vi "SimpleRegAndResolve.vi"() -> ()   [LabVIEW 2024, in "Module Container.lvlib"]
uses:
  Module Container.lvlib
  ModuleTemplates/NewTemplateModule/NewTemplate.lvclass
  C:/Git/JA/JQMH/RQMHCore/ModuleCore/Module.lvclass
  C:/Git/JA/JQMH/ModuleTemplates/NewTemplateModule/NewTemplate.lvclass
  ModuleCore/Module.lvclass
  Startup/ModuleStartup.lvclass
panel:
  out "Already Running":bool
  out "error out":errorcluster
  in  "stop":bool
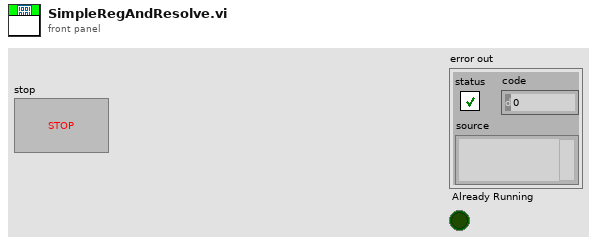
[diagram p1: front panel]
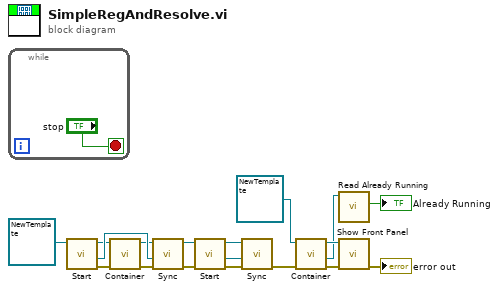
[diagram p0: block diagram]
diagram:
  n1 = while {
    stop <- "stop" stop-if-true
  }
  n2 = call "Start.vi"("JQMHCore in"=refnum<class "NewTemplate.lvclass"> refnum ("Template")) -> ("error out"=w9:errorcluster, "StartupHandshake out"=w18:refnum<class "ModuleStartup.lvclass">, "JQMHCore out"=w13:refnum<class "NewTemplate.lvclass">)  [unwired: 8 in]
  n3 = call "Container.vi"("error in (no error)"=w9, "Module Type"=w13) -> ("error out"=w8:errorcluster, "Module Instance"=w12:refnum<class "NewTemplate.lvclass">)  [unwired: 7 in, 1 out]
  n4 = call "Sync.vi"("error in (no error)"=w8, "StartupHandshake out"=w18, "JQMHCore in"=w12) -> ("error out"=w7:errorcluster, "JQMHCore out"=w16:refnum<class "NewTemplate.lvclass">)  [unwired: 7 in]
  n5 = call "Start.vi"("error in (no error)"=w7, "JQMHCore in"=w16) -> ("error out"=w17:errorcluster, "StartupHandshake out"=w14:refnum<class "ModuleStartup.lvclass">, "JQMHCore out"=w15:refnum<class "NewTemplate.lvclass">)  [unwired: 7 in]
  n6 = call "Sync.vi"("error in (no error)"=w17, "StartupHandshake out"=w14, "JQMHCore in"=w15) -> ("error out"=w11:errorcluster)  [unwired: 7 in, 1 out]
  n7 = call "Container.vi"("error in (no error)"=w11, "Module Type"=refnum<class "NewTemplate.lvclass"> refnum ("Template")) -> ("error out"=w6:errorcluster, "Handshake (if started)"=w4:refnum<class "ModuleStartup.lvclass">, "Module Instance"=w10:refnum<class "NewTemplate.lvclass">)  [unwired: 7 in]
  n8 = call "Read Already Running.vi"("JQMHStartup in"=w4) -> ("Already Running"=→"Already Running":bool)  [unwired: 9 in, 1 out]
  n9 = call "Show Front Panel.vi"("error in (no error)"=w6, "JQMHCore in"=w10) -> ("error out"=→"error out":errorcluster)  [unwired: 8 in, 1 out]
